vi "TestExec.Config, Get Station Module Dock State.vi"() -> (3 "Dock?":bool)   [LabVIEW 2018]
uses:
  <vilib>/Utility/config.llb/Read Key (String).vi
  <vilib>/Utility/config.llb/NI_LVConfig.lvlib
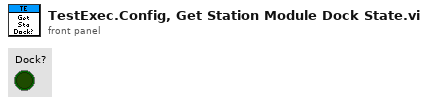
[diagram p1: front panel]
types:
  T1 = enum32{"invalid app kind", "Development System", "Run Time System", "Student Edition", "Embedded LabVIEW", "Evaluation", "Custom"}
  T2 = typedef "NI_LVConfig.lvlib/Config Data RefNum.ctl" = refnum<k1>
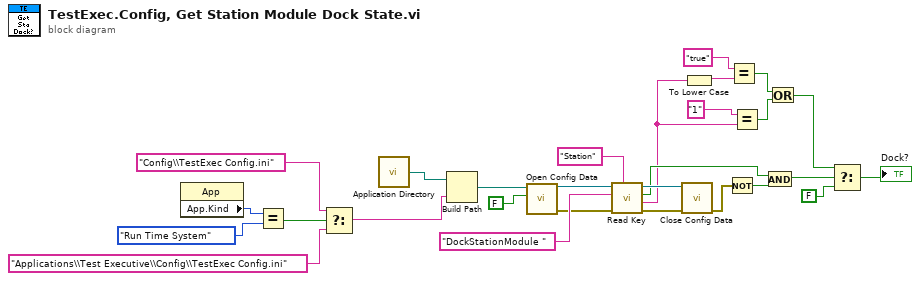
[diagram p0: block diagram]
diagram:
  n1 = property class="App"() -> ("App.Kind"=w16:T1)  [unwired: 2 in, 2 out]
  n2 = Equal?(x=w16, y=T1."Run Time System" ("Application:Kind")) -> (x = y?=w12:bool)
  n3 = Select(t="Config\\TestExec Config.ini", s=w12, f="Applications\\Test Executive\\Config\\TestExec Config.ini") -> (s? t:f=w11:string)
  n4 = call <vilib>:"Application Directory.vi"() -> ("Application Directory"=w18:path)
  n5 = Build Path(base path=w18, name or relative path=w11) -> (appended path=w17:path)
  n6 = call <vilib>:"Open Config Data.vi"("create file if necessary (T)"=FALSE, "configuration file path"=w17) -> ("error out"=w25:errorcluster, "refnum"=w28:T2)  [unwired: 7 in, 1 out]
  n7 = call-poly <vilib>:"Read Key.vi"("section"="Station", "error in (no error)"=w25, "key"="DockStationModule ", "refnum"=w28) -> ("error out"=w22:errorcluster, "value"=w4:string, "found?"=w19:bool, "refnum out"=w23:T2)  [unwired: 4 in]
  n8 = call <vilib>:"Close Config Data.vi"("error in (no error)"=w22, "refnum"=w23) -> ("error out"=w20:errorcluster)  [unwired: 8 in, 1 out]
  n9 = To Lower Case(string=w4) -> (all lower case string=w6:string)
  n10 = Not(x=w20) -> (.not. x?=w21:bool)
  n11 = Equal?(x="true", y=w6) -> (x = y?=w2:bool)
  n12 = Equal?(x="1", y=w4) -> (x = y?=w3:bool)
  n13 = And(x=w19, y=w21) -> (x .and. y?=w10:bool)
  n14 = Or(x=w2, y=w3) -> (x .or. y?=w1:bool)
  n15 = Select(t=w1, s=w10, f=FALSE) -> (s? t:f=→"Dock?":bool)
